vi "OnCollision.vi"(7 "Game in":refnum<class "Game.lvclass">, 8 "error in (no error)":errorcluster, 9 "Engine in":refnum<class "Engine.lvclass">, 10 "Collider":refnum<class "GameObject.lvclass">, 11 "BounceTarget in":refnum<class "BounceTarget.lvclass">) -> (0 "error out":errorcluster, 1 "Engine out":refnum<class "Engine.lvclass">, 2 "Colliderout":refnum<class "GameObject.lvclass">, 3 "BounceTarget out":refnum<class "BounceTarget.lvclass">, 5 "Game out":refnum<class "Game.lvclass">)   [LabVIEW 2019, in "RT_Game.lvlib" / "BounceTarget.lvclass"]
uses:
  BounceTarget.lvclass
  C:/Users/FreshBob/Dropbox/VIs/myRIO_GameConsole/RT/RT_Game/GameObject/GameObject.lvclass
  GameObject/GameObject.lvclass
  Game/Game.lvclass
  Engine/Engine.lvclass
  BounceTarget.lvclass/BounceTarget.ctl
  GameObject/GameObject.lvclass/GameObject.ctl
  GameObject/Write IsActive.vi
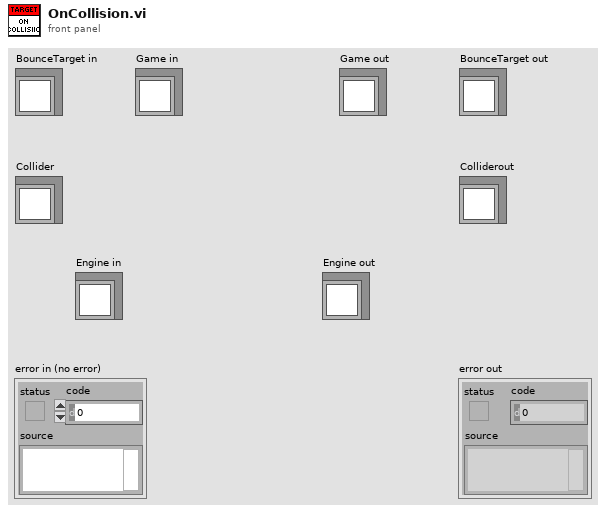
[diagram p1: front panel]
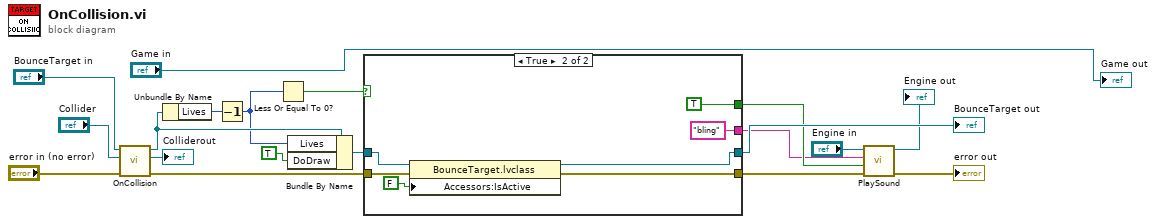
[diagram p0: block diagram]
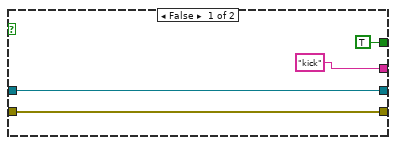
[diagram p2: hidden frame]
diagram:
  n1 = call-parent "OnCollision.vi"("error in (no error)"="error in (no error)", "Collider"="Collider", "GameObject in"="BounceTarget in") -> ("error out"=w19:errorcluster, "Colliderout"=→"Colliderout":refnum<class "GameObject.lvclass">, "GameObject out"=w14:refnum<class "BounceTarget.lvclass">)  [unwired: 4 in, 2 out]
  n2 = Unbundle By Name(w14) -> ("Lives"=w12:i16)
  n3 = Decrement(x=w12) -> (x-1=w11:i16)
  n4 = Less Or Equal To 0?(x=w11) -> (x <= 0?=w10:bool)
  n5 = Bundle By Name(cluster=w14, "Lives"=w11, "DoDraw"=TRUE) -> (w13:refnum<class "BounceTarget.lvclass">)
  n6 = case shown="True" w10 {
    tunnel: w19 -> [w22 w30]
    tunnel: [w22 w29] -> w15
    tunnel: [w23 w28] -> w6
    tunnel: w13 -> [w23 w26]
    tunnel: [TRUE ("Overwrite? (T)") TRUE ("Overwrite? (T)")] -> w5
    tunnel: ["kick" ("Name") "bling" ("Name")] -> w4
    frame False {
    }
    frame True {
      n7 = property class="BounceTarget.lvclass"(reference=w26, error in=w30, "Accessors:IsActive"=FALSE ("IsActive")) -> (reference out=w28:refnum<class "BounceTarget.lvclass">, error out=w29:errorcluster)
    }
  }
  "BounceTarget out" <- w6
  n8 = call "PlaySound.vi"("error in (no error)"=w15, "Overwrite"=w5, "Name"=w4, "Engine in"="Engine in") -> ("error out"=→"error out":errorcluster, "Engine out"=→"Engine out":refnum<class "Engine.lvclass">)  [unwired: 6 in]
  "Game out" <- "Game in"
